vi "Read_angle.vi"(8 "error in (no error)":errorcluster, 11 "Task cluster In":T1) -> (0 "error out":errorcluster, 1 "Found index?":bool, 2 "appended array":dbl[](array[numeric]), 3 "Task cluster Out":T1)   [LabVIEW 2018, in "Motor_ReadAng.lvlib"]
doc: "Takes the encoder clusters as inputs and processes them to geenrate angles in degrees bounded between -180 to +180.\n\nRemember to open the tasks before reading and also stop the tasks when done!"
uses:
  Motor_ReadAng.lvlib
  Task cluster.ctl
  <vilib>/DAQmx/read.llb/DAQmx Read (Digital Bool 1Line 1Point).vi
  <vilib>/DAQmx/read.llb/DAQmx Read (Counter DBL 1Chan 1Samp).vi
  <vilib>/DAQmx/miscellaneous.llb/DAQmx Fill In Error Info.vi
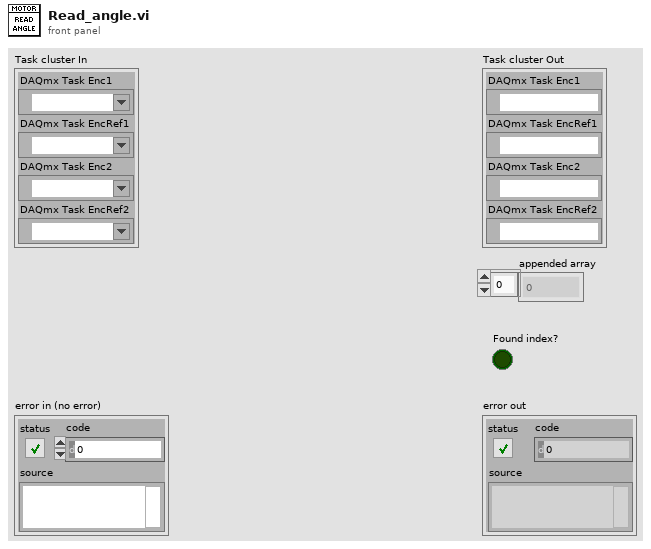
[diagram p1: front panel]
types:
  T1 = typedef "Motor_ReadAng.lvlib/Task cluster.ctl" = cluster{"DAQmx Task Enc1":refnum<k21>, "DAQmx Task EncRef1":refnum<k21>, "DAQmx Task Enc2":refnum<k21>, "DAQmx Task EncRef2":refnum<k21>}
  T2 = enum16{"Rising Edge", "Falling Edge", "Any Edge"}
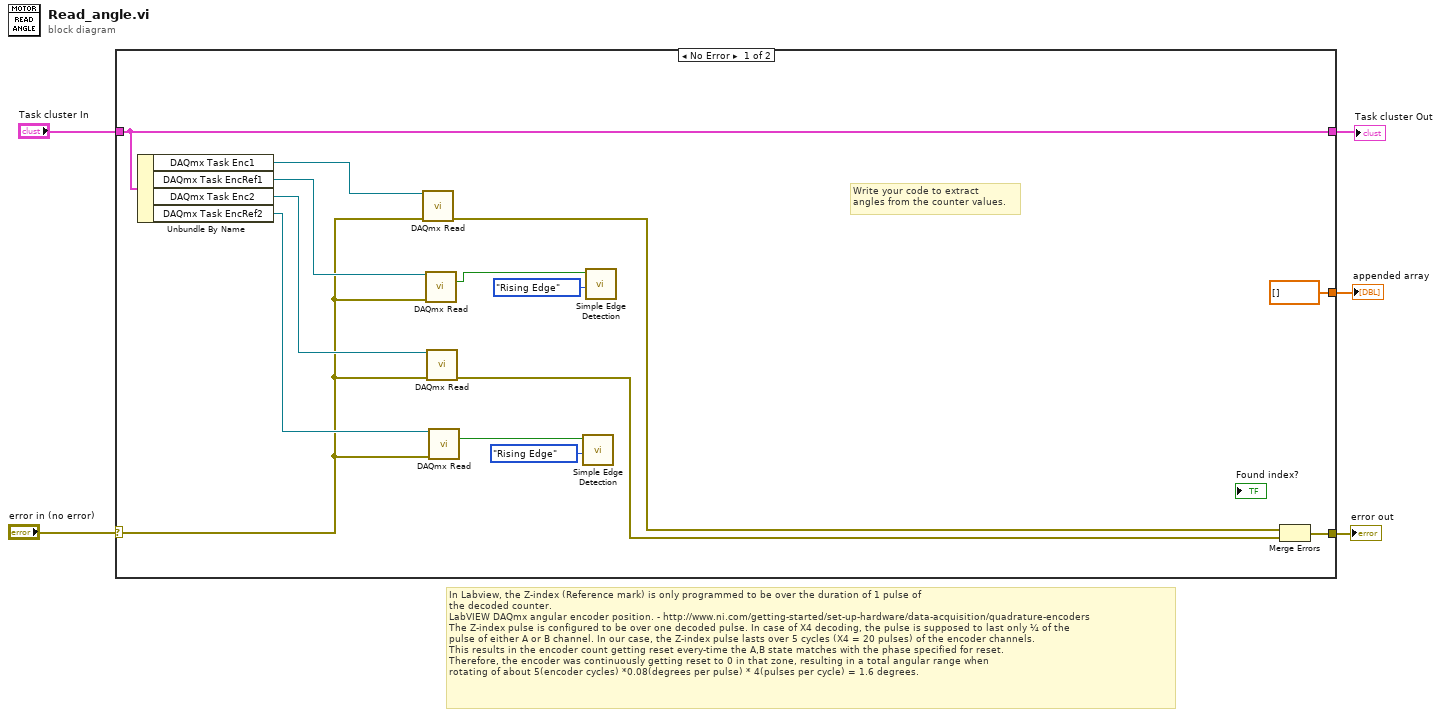
[diagram p0: block diagram]
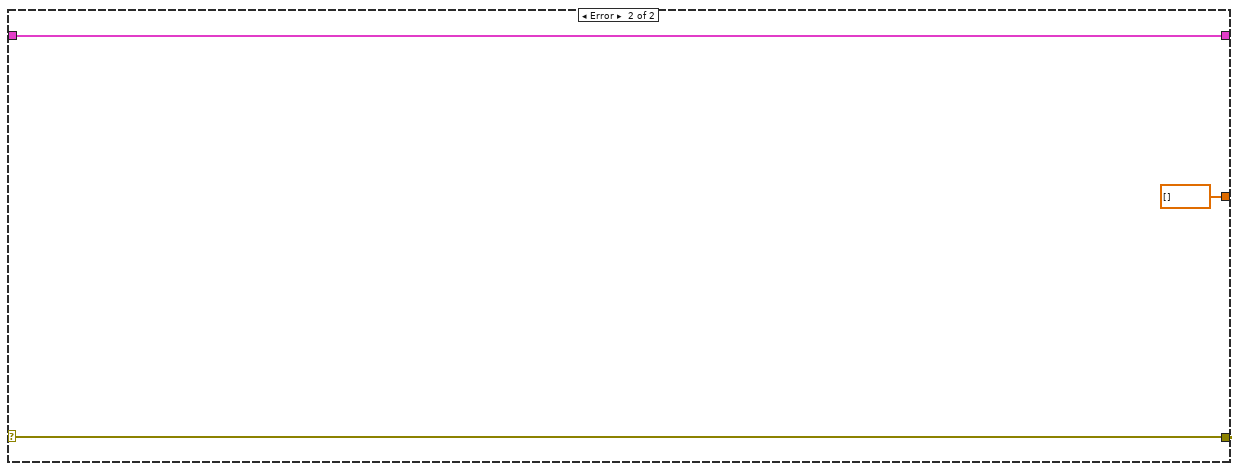
[diagram p2: hidden frame]
diagram:
  # "In Labview, the Z-index (Reference mark) is only programmed to be over the duration of 1 pulse of\nthe decoded counter.\nLabVIEW DAQmx angular encoder position. - http://www.ni.com/getting-started/set-up-hardware/data-acquisition/quadrature-encoders\nThe Z-index pulse is configured to be over one decoded pulse. In case of X4 decoding, the pulse is supposed to last only ¼ of the\npulse of either A or B channel. In our case, the Z-index pulse lasts over 5 cycles (X4 = 20 pulses) of the encoder channels. \nThis results in the encoder count getting reset every-time the A,B state matches with the phase specified for reset. \nTherefore, the encoder was continuously getting reset to 0 in that zone, resulting in a total angular range when \nrotating of about 5(encoder cycles) *0.08(degrees per pulse) * 4(pulses per cycle) = 1.6 degrees."
  n1 = case shown="No Error" "error in (no error)" {
    selector: "error in (no error)" -> [w14 w22]
    tunnel: [w13 w22] -> w4
    tunnel: "Task cluster In" -> [w19 w21]
    tunnel: [w19 w21] -> w2
    tunnel: [dbl[] [] dbl[] []] -> w1
    frame No Error {
      # "Write your code to extract \nangles from the counter values."
      n2 = Unbundle By Name(w19) -> ("DAQmx Task Enc1"=w18:refnum<k21>, "DAQmx Task EncRef1"=w17:refnum<k21>, "DAQmx Task Enc2"=w16:refnum<k21>, "DAQmx Task EncRef2"=w15:refnum<k21>)
      n3 = call-poly <vilib>:"DAQmx Read.vi"("task/channels in"=w18, "error in"=w14) -> ("error out"=w8:errorcluster)  [unwired: 11 in, 2 out]
      n4 = call-poly <vilib>:"DAQmx Read.vi"("task/channels in"=w17, "error in"=w14) -> ("data"=w12:bool)  [unwired: 11 in, 2 out]
      n5 = call-poly <vilib>:"DAQmx Read.vi"("task/channels in"=w16, "error in"=w14) -> ("error out"=w7:errorcluster)  [unwired: 11 in, 2 out]
      n6 = call-poly <vilib>:"DAQmx Read.vi"("task/channels in"=w15, "error in"=w14) -> ("data"=w9:bool)  [unwired: 11 in, 2 out]
      n7 = call "Simple Edge Detection.vi"("Mode"=T2."Rising Edge", "clk_in"=w9) -> ()  [unwired: 9 in, 1 out]
      n8 = call "Simple Edge Detection.vi"("Mode"=T2."Rising Edge", "clk_in"=w12) -> ()  [unwired: 9 in, 1 out]
      n9 = Merge Errors(w8, w7) -> (w13:errorcluster)
    }
    frame Error {
    }
  }
  "error out" <- w4
  "Task cluster Out" <- w2
  "appended array" <- w1
